vi "Find Actor Core.vi"() -> (1 "Actor Core VI Name":string, 2 "Found":bool)   [LabVIEW 2018, in "Monitored Actor.lvlib" / "Monitored Actor.lvclass"]
doc: "Looks through the call chain to find the correct version of actor core. We the Child's specific implementation of actor core if possible.\n\nBecause this will look through the call chain, this VI only works if it's run in a do method of an actor. (Not in pre-launch init for example)\n\nCopyright: Hill AFB\nAuthored By: Derek Trepanier"
uses:
  Monitored Actor.lvclass
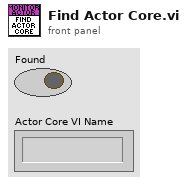
[diagram p1: front panel]
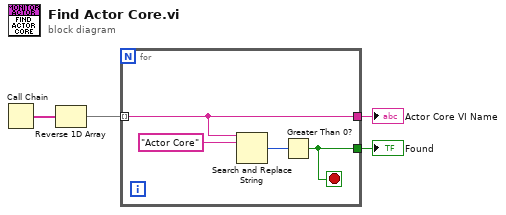
[diagram p0: block diagram]
diagram:
  n1 = Call Chain() -> (call chain=w1:string[])
  n2 = Reverse 1D Array(array=w1) -> (reversed array=w2:string[])
  n3 = for {
    tunnel: w2 -> [w5] mode=indexing
    tunnel: [w6] -> w3
    tunnel: [w5] -> w4
    stop <- w6 stop-if-true
    n4 = Search and Replace String(input string=w5, search string="Actor Core") -> (number of replacements=w7:i32)  [unwired: 6 in, 3 out]
    n5 = Greater Than 0?(x=w7) -> (x > 0?=w6:bool)
  }
  "Actor Core VI Name" <- w4
  "Found" <- w3
